vi "Unindent.vi"(1 "Line String":string) -> (0 "Index":u32)   [LabVIEW 2015, in "YAML Parser.lvclass"]
uses:
  YAML Parser.lvclass
  <vilib>/regexp/Match Regular Expression.xnode
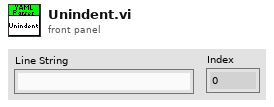
[diagram p1: front panel]
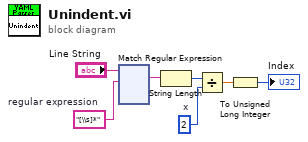
[diagram p0: block diagram]
diagram:
  w2 = 2  # x
  w6 = "[\\s]*"  # regular expression
  n1 = xnode "Match Regular Expression"("input string"="Line String", "regular expression"=w6) -> ("whole match"=w5:string)  [unwired: 4 in, 4 out]
  n2 = String Length(string=w5) -> (length=w4:i32)
  n3 = Divide(x=w4, y=w2) -> (x/y=w3:dbl)
  n4 = To Unsigned Long Integer(number=w3) -> (unsigned 32bit integer=→"Index":u32)
